vi "Open Front Panel.vi"(8 "error in (no error)":errorcluster, 11 "ViewableActor in":refnum<class "ViewableActor.lvclass">) -> (0 "error out":errorcluster, 3 "ViewableActor out":refnum<class "ViewableActor.lvclass">)   [LabVIEW 2020, in "ViewableActor.lvlib" / "ViewableActor.lvclass"]
uses:
  ViewableActor.lvclass
  ViewableActor.lvclass/ViewableActor.ctl
  Read UI VI Ref.vi
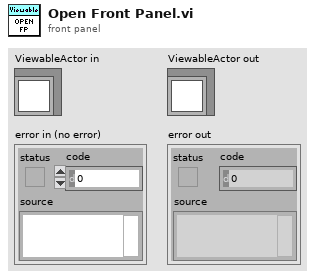
[diagram p1: front panel]
types:
  T1 = enum32{"Invalid", "Standard", "Closed", "Hidden", "Minimized", "Maximized"}
  T2 = typedef "LVRectTypeDef.ctl" = cluster{"Left":i16, "Top":i16, "Right":i16, "Bottom":i16}
  T3 = cluster{"Left":bool, "Top":bool, "Right":bool, "Bottom":bool}
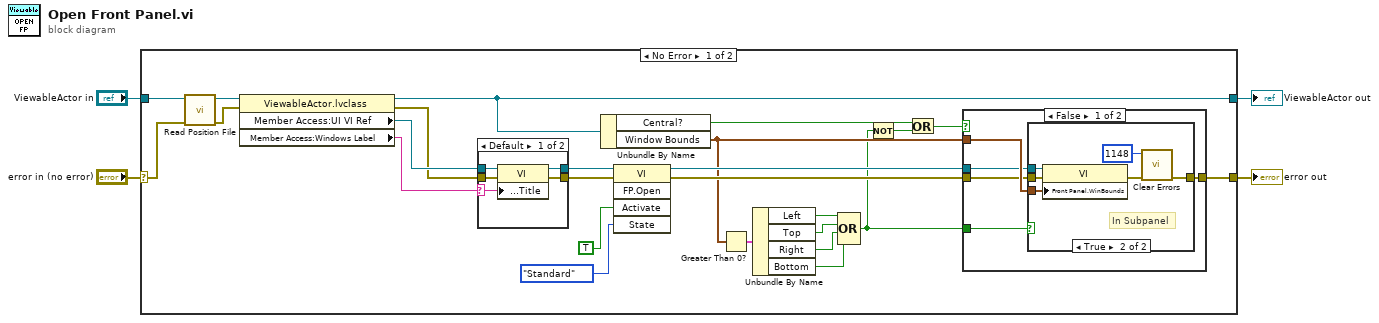
[diagram p0: block diagram]
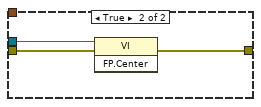
[diagram p3: hidden frame]
diagram:
  n1 = case shown="No Error" "error in (no error)" {
    selector: "error in (no error)" -> [w6 w53]
    tunnel: [w18 w53] -> w3
    tunnel: [w21 w52] -> w1
    tunnel: "ViewableActor in" -> [w29 w52]
    frame No Error {
      n2 = call "Read Position File.vi"("error in (no error)"=w6, "ViewableActor in"=w29) -> ("error out"=w5:errorcluster, "ViewableActor out"=w7:refnum<class "ViewableActor.lvclass">)  [unwired: 8 in]
      n3 = property class="ViewableActor.lvclass"(reference=w7, error in=w5) -> (reference out=w21:refnum<class "ViewableActor.lvclass">, error out=w24:errorcluster, "Member Access:UI VI Ref"=w28:refnum<vi>, "Member Access:Windows Label"=w22:string)
      n4 = case shown="Default" w22 {
        selector: w22 -> [w45 _]
        tunnel: w28 -> [w49 w50]
        tunnel: [w48 w50] -> w25
        tunnel: w24 -> [w47 w51]
        tunnel: [w46 w51] -> w23
        frame Default {
          n5 = property class="VI"(reference=w49, error in=w47, "Front Panel.Title"=w45) -> (reference out=w48:refnum<vi>, error out=w46:errorcluster)
        }
        frame "" {
        }
      }
      n6 = Unbundle By Name(w21) -> ("Central?"=w17:bool, "Window Bounds"=w11:T2)
      n7 = invoke class="VI" method="FP.Open"(reference=w25, error in=w23, "Activate"=TRUE ("Activate?"), "State"=T1."Standard") -> (reference out=w20:refnum<vi>, error out=w19:errorcluster)  [unwired: 1 in, 3 out]
      n8 = Greater Than 0?(x=w11) -> (x > 0?=w12:T3)
      n9 = Unbundle By Name(w12) -> ("Left"=w13:bool, "Top"=w14:bool, "Right"=w15:bool, "Bottom"=w16:bool)
      n10 = Compound Arithmetic op=OR(w13, w14, w15, w16) -> (w9:bool)
      n11 = Not(x=w9) -> (.not. x?=w8:bool)
      n12 = Or(x=w17, y=w8) -> (x .or. y?=w10:bool)
      n13 = case shown="False" w10 {
        tunnel: w20 -> [w33 w44]
        tunnel: w19 -> [w32 w43]
        tunnel: [w31 w42] -> w18
        tunnel: w11 -> [w34 _]
        tunnel: w9 -> [w30 _]
        frame False {
          n14 = case shown="True" w30 {
            tunnel: w32 -> [w35 w41]
            tunnel: [w35 w37] -> w31
            tunnel: w33 -> [_ w39]
            tunnel: w34 -> [_ w38]
            frame False {
            }
            frame True {
              # "In Subpanel"
              n15 = property class="VI"(reference=w39, error in=w41, "Front Panel.WinBounds"=w38) -> (error out=w40:errorcluster)  [unwired: 1 out]
              n16 = call <vilib>:"Clear Errors.vi"("error in (no error)"=w40, "specific error code to clear (0: all)"=1148) -> ("error out"=w37:errorcluster)  [unwired: 4 in, 1 out]
            }
          }
        }
        frame True {
          n17 = invoke class="VI" method="FP.Center"(reference=w44, error in=w43) -> (error out=w42:errorcluster)  [unwired: 1 in, 2 out]
        }
      }
    }
    frame Error {
    }
  }
  "error out" <- w3
  "ViewableActor out" <- w1
